vi "Convert Point 2D To Vertical ROI.vi"(10 "Vertical Delta":dbl, 11 "Point 2D":T2) -> (3 "ROI Descriptor":T1)   [LabVIEW 2015]
uses:
  Application Specific/Controls/Point 2D.ctl
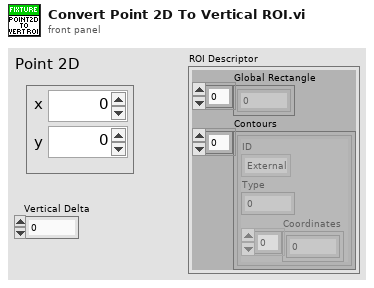
[diagram p1: front panel]
types:
  T1 = cluster{"Global Rectangle":i32[], "Contours":cluster{"ID":enum32{"External", "Internal"}, "Type":u32, "Coordinates":i32[]}[]}
  T2 = typedef "Point 2D.ctl" = cluster{"x":dbl, "y":dbl}
  T3 = cluster{"ID":enum32{"External", "Internal"}, "Type":u32, "Coordinates":i32[]}
  T4 = cluster{"ID":enum32{"External", "Internal"}, "Type":u32, "Coordinates":i32[]}[]
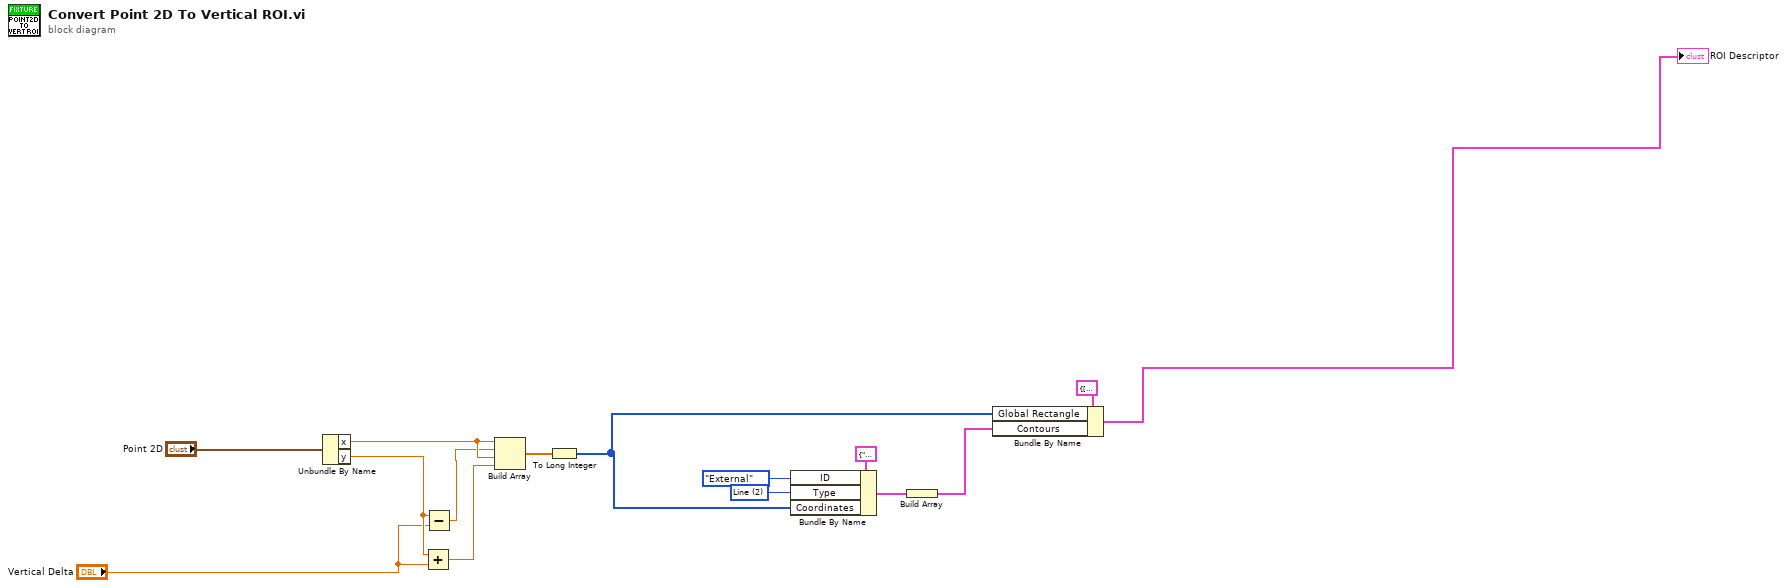
[diagram p0: block diagram]
diagram:
  w3 = u32 2 items=["No Selection", "Point", "Line", "Rectangle", "Oval", "Polygon", "Freehand Region", "Annulus", "Unused2", "Unused3", "Broken Line", "Freehand Line", "Rotated Rectangle"] ("Type")
  n1 = Unbundle By Name("Point 2D") -> ("x"=w8:dbl, "y"=w6:dbl)
  n2 = Add(x=w6, y="Vertical Delta") -> (x+y=w5:dbl)
  n3 = Subtract(x=w6, y="Vertical Delta") -> (x-y=w7:dbl)
  n4 = Build Array(w8, w7, w8, w5) -> (w9:dbl[])
  n5 = To Long Integer(number=w9) -> (32bit integer=w12:i32[])
  n6 = Bundle By Name(cluster=T3 {"ID"=enum."External", "Type"=2, "Coordinates"=[20, 39, 20, 21]}, "ID"=enum32{"External", "Internal"}."External", "Type"=w3, "Coordinates"=w12) -> (w10:T3)
  n7 = Build Array(w10) -> (w11:T4)
  n8 = Bundle By Name(cluster=T1 {"Global Rectangle"=[20, 21, 21, 40], "Contours"=[{"ID"=enum."Internal", "Type"=2, "Coordinates"=[20, 39, 20, 21]}]} ("ROI Descriptor"), "Global Rectangle"=w12, "Contours"=w11) -> (→"ROI Descriptor":T1)
